vi "Main.vi"() -> ()   [LabVIEW 2015]
doc: "This template is for the Queued Message Handler design pattern.\n\nThe Event Handling Loop generates messages based on user interface actions.\n\nThe Message Handling Loop processes messages generated by the Event Handling Loop, or by other messages. The messages are string values, so new messages can be added easily to the Message Cases case structure in the Message Handling Loop. Each message cluster can also provide an optional value for Message Data, which is a variant that can be converted to whatever message-specific data is required."
uses:
  controls/UI Data.ctl
  support/Boiler System Globals.vi
  support/Message Queue/Message Queue.lvlib
  support/User Event - Stop/User Event - Stop.lvlib
panel:
  out "Display <Replace Me>":string
  in  "Do Something Else <Replace Me>":bool
  in  "Do Something <Replace Me>":bool
  in  "Stop Button":bool
  # "These controls have associated \"Value Changed\" events configured in the Event Structure on the diagram.\n\nReplace them (and reconfigure the Event Structure) with the controls you need for your application."
  # "This template is for the Queued Message Handler design pattern.\n\nSee the block diagram for more information on how to use this template."
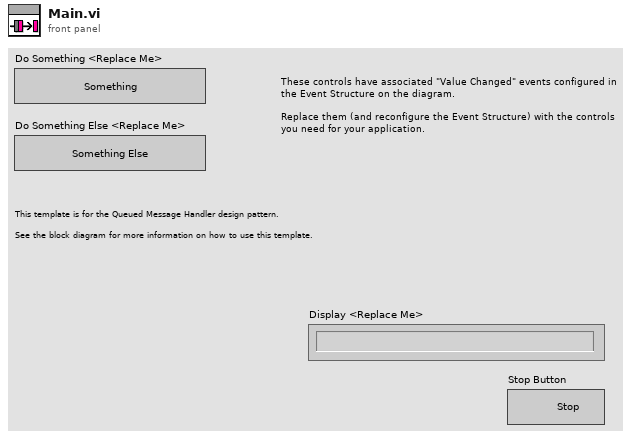
[diagram p1: front panel]
types:
  T1 = typedef "UI Data.ctl" = cluster{"Boolean <Replace Me>":bool, "String <Replace Me>":string, "Numeric <Replace Me>":dbl, "Do Something Ref":refnum<vi>, "Do Something Else Ref":refnum<vi>, "Data Display Ref":refnum<vi>, "Stop Button Ref":refnum<vi>}
  T2 = typedef "Message Queue.lvlib/All Message Queues.ctl" = cluster{"MHL":refnum<queue>, "Boiler Controller":refnum<queue>}
  T3 = enum32{"invalid app kind", "Development System", "Run Time System", "Student Edition", "Embedded LabVIEW", "Evaluation", "Custom"}
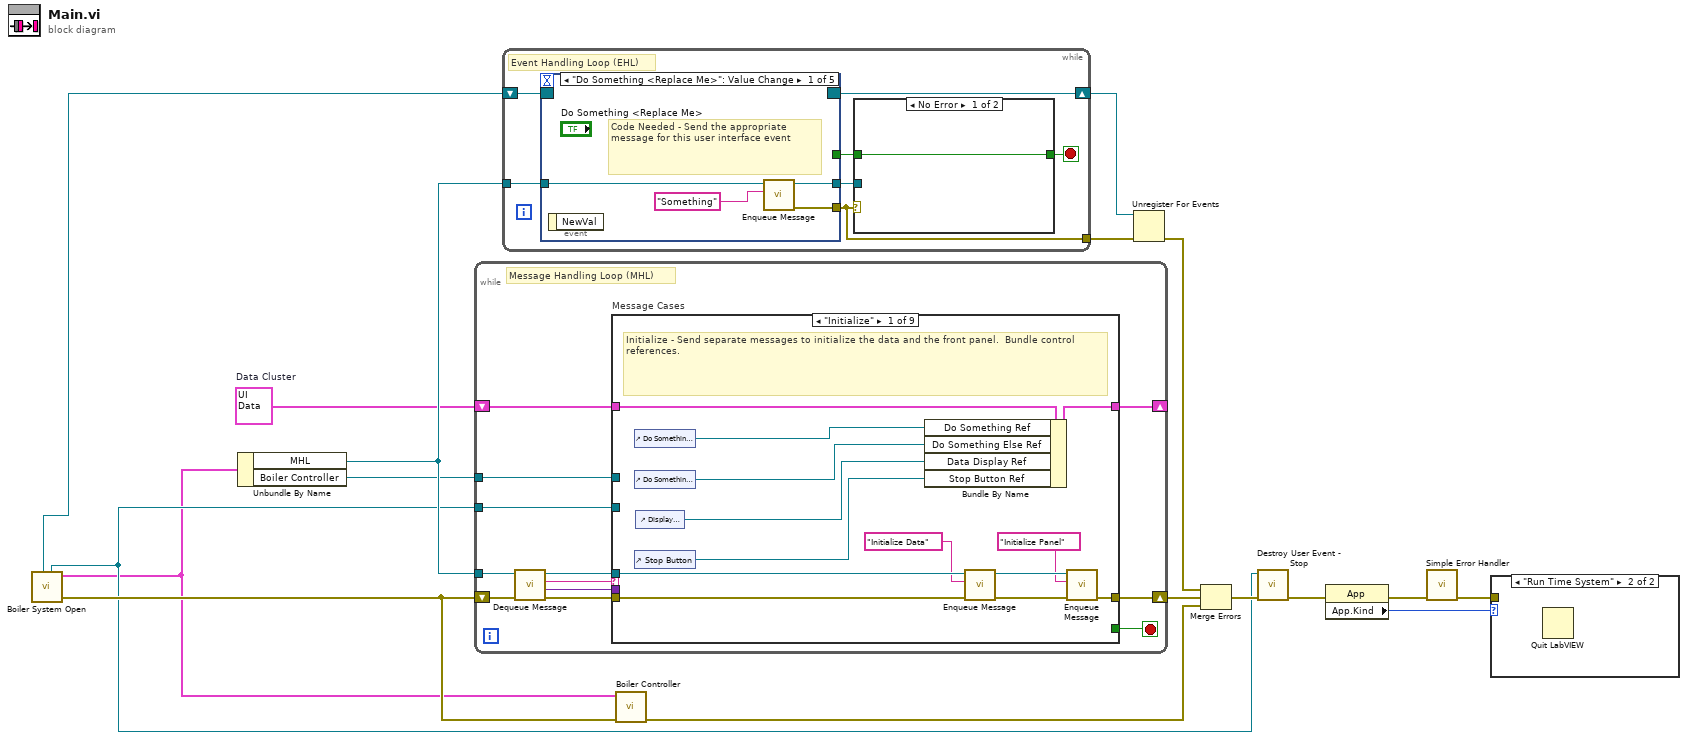
[diagram p0: block diagram]
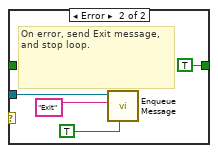
[diagram p3: hidden frame]
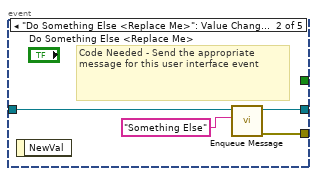
[diagram p4: hidden frame]
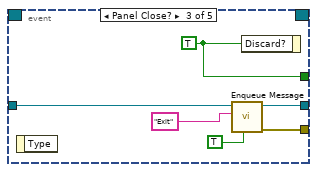
[diagram p5: hidden frame]
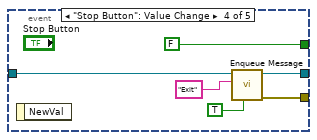
[diagram p6: hidden frame]
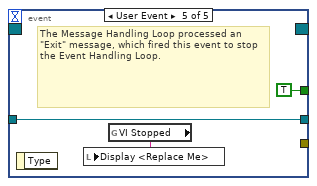
[diagram p7: hidden frame]
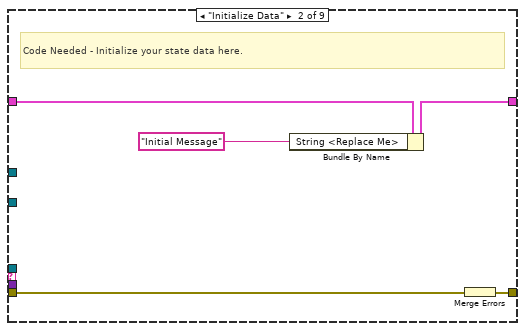
[diagram p8: hidden frame]
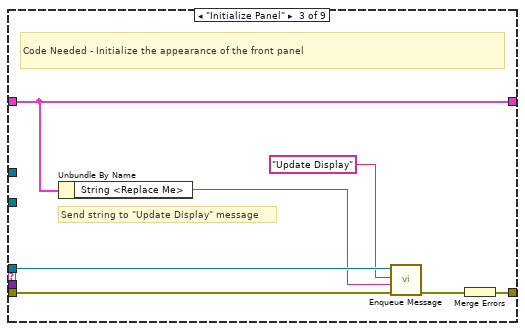
[diagram p9: hidden frame]
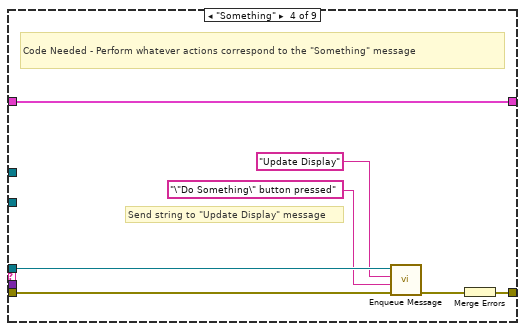
[diagram p10: hidden frame]
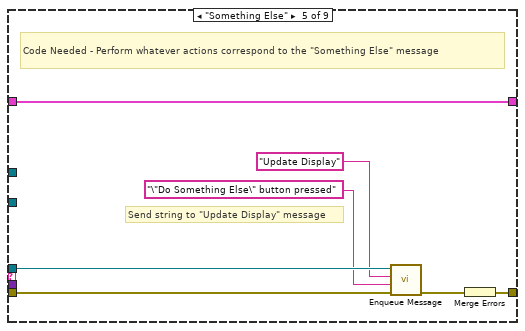
[diagram p11: hidden frame]
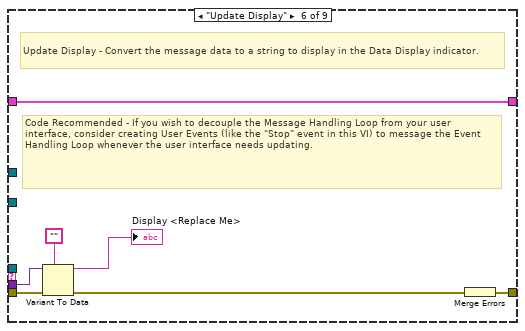
[diagram p12: hidden frame]
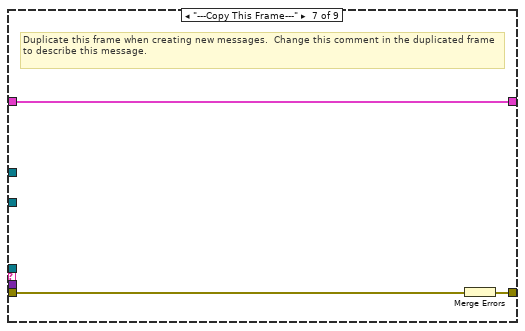
[diagram p13: hidden frame]
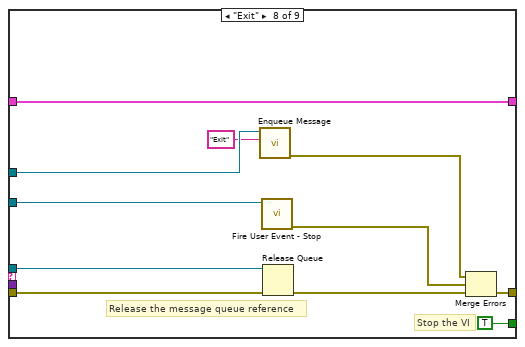
[diagram p14: hidden frame]
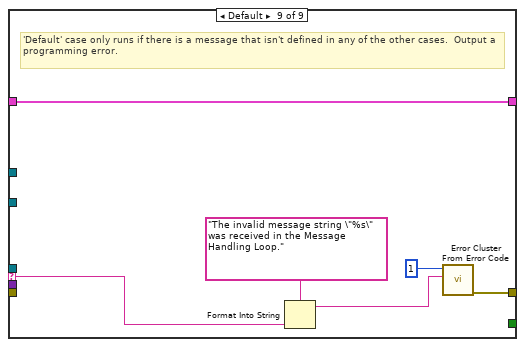
[diagram p15: hidden frame]
diagram:
  w10 = T1 {"Boolean <Replace Me>"=TRUE, "String <Replace Me>"="", "Numeric <Replace Me>"=0.0, "Do Something Ref"=refnum, "Do Something Else Ref"=refnum, "Data Display Ref"=refnum, "Stop Button Ref"=refnum}  # Data Cluster
  n1 = call "Boiler System Open.vi"() -> ("error out"=w4:errorcluster, "Message Queues out"=w1:T2, "User Event - Stop"=w2:refnum<user-event>, "Stop Event Registration Refnum"=w3:refnum<event-registration>)  [unwired: 7 in, 1 out]
  n2 = Unbundle By Name(w1) -> ("MHL"=w16:refnum<queue>, "Boiler Controller"=w8:refnum<queue>)
  n3 = while {
    tunnel: w16 -> [w19]
    shift-right: [w28] -> _
    shift-left: w10 -> [w29]
    tunnel: w2 -> [w25]
    shift-right: [w26] -> w17
    shift-left: w4 -> [w24]
    tunnel: w8 -> [w18]
    stop <- w27 stop-if-true
    # "Message Handling Loop (MHL)"
    n4 = call "Dequeue Message.vi"("error in (no error)"=w24, "Message Queue"=w19) -> ("error out"=w23:errorcluster, "Message Data"=w21:variant, "Message"=w22:string, "dup Message Queue"=w20:refnum<queue>)  [unwired: 6 in]
    n5 = case "Message Cases" shown="\"Initialize\"" w22 {
      selector: w22 -> [_ _ _ _ _ _ _ _ w93]
      tunnel: w20 -> [w38 _ w51 w57 w64 _ _ w89 _]
      tunnel: w23 -> [w41 w47 w52 w59 w66 w73 w78 w80 _]
      tunnel: [w42 w43 w53 w60 w67 w74 w76 w85 w91] -> w26
      tunnel: w29 -> [w35 w46 w54 w61 w68 w75 w77 w88 w95]
      tunnel: [w34 w45 w54 w61 w68 w75 w77 w88 w95] -> w28
      tunnel: [_ _ _ _ _ _ _ TRUE _] -> w27
      tunnel: w21 -> [_ _ _ _ _ w72 _ _ _]
      tunnel: w25 -> [_ _ _ _ _ _ _ w84 _]
      tunnel: w18 -> [_ _ _ _ _ _ _ w82 _]
      frame "Initialize" {
        # "Initialize - Send separate messages to initialize the data and the front panel.  Bundle control references."
        n6 = control-ref of="Do Something <Replace Me>"() -> (w33:refnum<vi>)
        n7 = control-ref of="Do Something Else <Replace Me>"() -> (w32:refnum<vi>)
        n8 = control-ref of="Stop Button"() -> (w30:refnum<vi>)
        n9 = control-ref of="Display <Replace Me>"() -> (w31:refnum<vi>)
        n10 = Bundle By Name(cluster=w35, "Do Something Ref"=w33, "Do Something Else Ref"=w32, "Data Display Ref"=w31, "Stop Button Ref"=w30) -> (w34:T1)
        n11 = call "Enqueue Message.vi"("error in (no error)"=w41, "Message"="Initialize Data", "Message Queue"=w38) -> ("error out"=w40:errorcluster, "dup Message Queue"=w39:refnum<queue>)  [unwired: 7 in]
        n12 = call "Enqueue Message.vi"("error in (no error)"=w40, "Message"="Initialize Panel", "Message Queue"=w39) -> ("error out"=w42:errorcluster)  [unwired: 7 in, 1 out]
      }
      frame "Initialize Data" {
        # "Code Needed - Initialize your state data here."
        n13 = Bundle By Name(cluster=w46, "String <Replace Me>"="Initial Message" ("Initial Message")) -> (w45:T1)
        n14 = Merge Errors(w47) -> (w43:errorcluster)
      }
      frame "Initialize Panel" {
        # "Send string to \"Update Display\" message"
        # "Code Needed - Initialize the appearance of the front panel"
        n15 = Unbundle By Name(w54) -> ("String <Replace Me>"=w48:string)
        n16 = call "Enqueue Message.vi"("error in (no error)"=w52, "Message Data"=w48, "Message"="Update Display", "Message Queue"=w51) -> ("error out"=w50:errorcluster)  [unwired: 6 in, 1 out]
        n17 = Merge Errors(w50) -> (w53:errorcluster)
      }
      frame "Something" {
        # "Send string to \"Update Display\" message"
        # "Code Needed - Perform whatever actions correspond to the \"Something\" message"
        n18 = call "Enqueue Message.vi"("error in (no error)"=w59, "Message Data"="\"Do Something\" button pressed" ("\"Do Something\" button pressed"), "Message"="Update Display", "Message Queue"=w57) -> ("error out"=w58:errorcluster)  [unwired: 6 in, 1 out]
        n19 = Merge Errors(w58) -> (w60:errorcluster)
      }
      frame "Something Else" {
        # "Send string to \"Update Display\" message"
        # "Code Needed - Perform whatever actions correspond to the \"Something Else\" message"
        n20 = call "Enqueue Message.vi"("error in (no error)"=w66, "Message Data"="\"Do Something Else\" button pressed" ("\"Do Something Else\" button pressed"), "Message"="Update Display", "Message Queue"=w64) -> ("error out"=w65:errorcluster)  [unwired: 6 in, 1 out]
        n21 = Merge Errors(w65) -> (w67:errorcluster)
      }
      frame "Update Display" {
        # "Code Recommended - If you wish to decouple the Message Handling Loop from your user interface, consider creating User Events (like the \"Stop\" event in this VI) to message the Event Handling Loop whenever the user interface needs updating."
        # "Update Display - Convert the message data to a string to display in the Data Display indicator."
        n22 = Variant To Data(error in=w73, type="", Variant=w72) -> (data=→"Display <Replace Me>":string, error out=w70:errorcluster)
        n23 = Merge Errors(w70) -> (w74:errorcluster)
      }
      frame "---Copy This Frame---" {
        # "Duplicate this frame when creating new messages.  Change this comment in the duplicated frame to describe this message."
        n24 = Merge Errors(w78) -> (w76:errorcluster)
      }
      frame "Exit" {
        # "Stop the VI"
        # "Release the message queue reference"
        n25 = call "Enqueue Message.vi"("Message"="Exit", "Message Queue"=w82) -> ("error out"=w79:errorcluster)  [unwired: 8 in, 1 out]
        n26 = call "Fire User Event - Stop.vi"("User Event - Stop"=w84) -> ("error out"=w83:errorcluster)  [unwired: 10 in]
        n27 = Release Queue(queue=w89, error in (no error)=w80) -> (error out=w86:errorcluster)  [unwired: 1 in, 2 out]
        n28 = Merge Errors(w79, w83, w86) -> (w85:errorcluster)
      }
      frame Default {
        # "'Default' case only runs if there is a message that isn't defined in any of the other cases.  Output a programming error."
        n29 = Format Into String(format string="The invalid message string \"%s\" was received in the Message Handling Loop." ("Unknown Message Error Text"), w93) -> (resulting string=w90:string)  [unwired: 2 in, 1 out]
        n30 = call <vilib>:"Error Cluster From Error Code.vi"("error message (\"\")"=w90, "error code (0)"=1) -> ("error out"=w91:errorcluster)  [unwired: 7 in]
      }
    }
  }
  n31 = while {
    tunnel: w16 -> [w102]
    tunnel: [w98] -> w12
    shift-right: [w96] -> w11
    shift-left: w3 -> [w97]
    stop <- w100 stop-if-true
    # "Event Handling Loop (EHL)"
    n32 = event shown="[0] \"Do Something <Replace Me>\": Value Change" {
      selector: w97 -> [_ _ _ _ _]
      dyn-events: [_ _ _ _ _] -> w96
      timeout: _ -> [_ _ _ _ _]
      tunnel: [_ _ w121 FALSE ("Discard?") TRUE ("Discard?")] -> w101
      tunnel: w102 -> [w111 w115 w120 w127 w130]
      tunnel: [w110 w113 w119 w126 _] -> w98
      tunnel: [w109 w114 w118 w124 w130] -> w99
      event "Do Something <Replace Me>": Value Change {
        # "Code Needed - Send the appropriate message for this user interface event"
        n33 = event-data() -> ()  [unwired: 1 in, 1 out]
        n34 = call "Enqueue Message.vi"("Message"="Something", "Message Queue"=w111) -> ("error out"=w110:errorcluster, "dup Message Queue"=w109:refnum<queue>)  [unwired: 8 in]
      }
      event "Do Something Else <Replace Me>": Value Change {
        # "Code Needed - Send the appropriate message for this user interface event"
        n35 = event-data() -> ()  [unwired: 1 in, 1 out]
        n36 = call "Enqueue Message.vi"("Message"="Something Else", "Message Queue"=w115) -> ("error out"=w113:errorcluster, "dup Message Queue"=w114:refnum<queue>)  [unwired: 8 in]
      }
      event Panel Close? {
        w121 = TRUE ("Discard?")
        n37 = event-data() -> ()  [unwired: 1 in, 1 out]
        n38 = call "Enqueue Message.vi"("Priority Message? (F)"=TRUE, "Message"="Exit", "Message Queue"=w120) -> ("error out"=w119:errorcluster, "dup Message Queue"=w118:refnum<queue>)  [unwired: 7 in]
        n39 = event-data("Discard?"=w121) -> ()  [unwired: 1 in, 1 out]
      }
      event "Stop Button": Value Change {
        n40 = event-data() -> ()  [unwired: 1 in, 1 out]
        n41 = call "Enqueue Message.vi"("Priority Message? (F)"=TRUE, "Message"="Exit", "Message Queue"=w127) -> ("error out"=w126:errorcluster, "dup Message Queue"=w124:refnum<queue>)  [unwired: 7 in]
      }
      event User Event {
        # "The Message Handling Loop processed an \"Exit\" message, which fired this event to stop the Event Handling Loop."
        n42 = event-data() -> ()  [unwired: 1 in, 1 out]
        n43 = global read "Boiler System Globals.vi" "VI Stopped"() -> (w128:string)
        n44 = local write "Display <Replace Me>"(w128) -> ()
      }
    }
    n45 = case shown="No Error" w98 {
      tunnel: [w103 TRUE ("Discard?")] -> w100
      tunnel: w101 -> [w103 _]
      tunnel: w99 -> [_ w106]
      frame No Error {
      }
      frame Error {
        # "On error, send Exit message, and stop loop."
        n46 = call "Enqueue Message.vi"("Priority Message? (F)"=TRUE, "Message"="Exit", "Message Queue"=w106) -> ()  [unwired: 7 in, 2 out]
      }
    }
  }
  n47 = call "Boiler Controller.vi"("error in"=w4, "Message Queues"=w1) -> ("error out"=w9:errorcluster)  [unwired: 9 in]
  n48 = Unregister For Events(event registration refnum=w11, error in=w12) -> (error out=w13:errorcluster)
  n49 = Merge Errors(w13, w17, w9) -> (w14:errorcluster)
  n50 = call "Destroy User Event - Stop.vi"("error in (no error)"=w14, "User Event - Stop"=w2) -> ("error out"=w15:errorcluster)  [unwired: 9 in]
  n51 = property class="App"(error in=w15) -> (error out=w7:errorcluster, "App.Kind"=w6:T3)  [unwired: 1 in, 1 out]
  n52 = call <vilib>:"Simple Error Handler.vi"("error in (no error)"=w7) -> ("error out"=w5:errorcluster)  [unwired: 4 in, 4 out]
  n53 = case shown="\"Run Time System\"" w6 {
    tunnel: w5 -> [_ _]
    frame Default {
    }
    frame "Run Time System" {
      n54 = Quit LabVIEW() -> ()  [unwired: 1 in]
    }
  }
